vi "vi.Array2Array.vi"(0 "Array":variant[](array[variant]), 11 "error in (no error)":errorcluster) -> (4 "ClusterArray":variant, 15 "error out":errorcluster)   [LabVIEW 2014, in "GLue.lvlib" / "class.GLue.lvclass"]
uses:
  class.GLue.lvclass
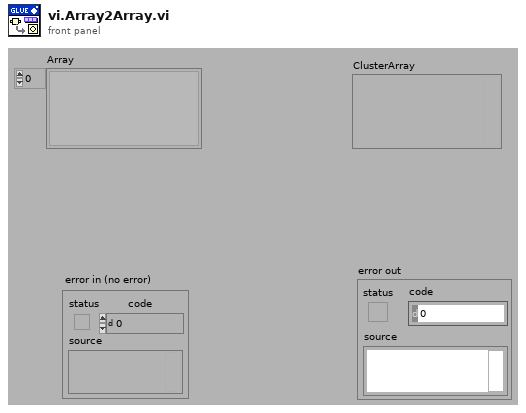
[diagram p1: front panel]
types:
  T1 = enum8{"<Null>", "I8", "I16", "I32", "I64", "U8", "U16", "U32", "U64", "SGL", "DBL", "EXT", "CSG", "CDB", "CXT", "0x0F", "0x10", "0x11", "0x12", "0x13", "0x14", "Enum U8", "Enum U16", "Enum U32", "Enum U64", "SGL PQ", "DBL PQ", "EXT PQ", "CSG PQ", "CDB PQ", "CXT PQ", "0x1F", "0x20", "Boolean", "0x22", "0x23", "0x24", "0x25", "0x26", "0x27", "0x28", "0x29", "0x2A", "0x2B", "0x2C", "0x2D", "0x2E", "0x2F", "String", "0x31", "Path", "Pict", "0x34", "0x35", "0x36", "DAQ", "0x38", "0x39", "0x3A", "0x3B", "0x3C", "0x3D", "0x3E", "0x3F", "Array", "0x41", "0x42", "0x43", "0x44", "0x45", "0x46", "0x47", "0x48", "0x49", "0x4A", "0x4B", "0x4C", "0x4D", "0x4E", "0x4F", "Cluster", "0x51", "0x52", "Variant", "Waveform", "0x55", "0x56", "0x57", "0x58", "0x59", "0x5A", "0x5B", "0x5C", "0x5D", "0x5E", "0x5F", "0x60", "0x61", "0x62", "0x63", "0x64", "0x65", "0x66", "0x67", "0x68", "0x69", "0x6A", "0x6B", "0x6C", "0x6D", "0x6E", "0x6F", "Refnum"}
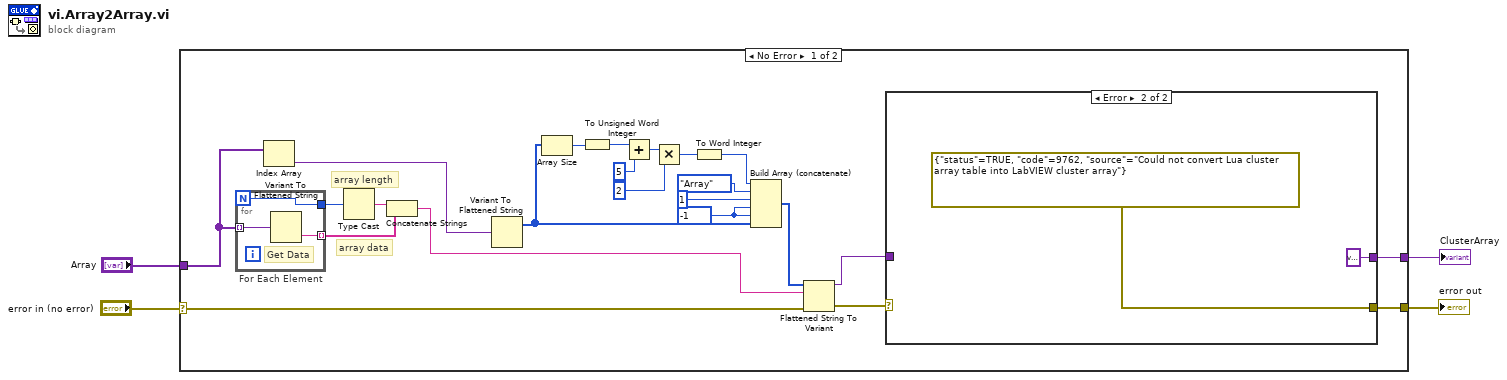
[diagram p0: block diagram]
diagram:
  n1 = case shown="No Error" "error in (no error)" {
    selector: "error in (no error)" -> [w9 w35]
    tunnel: "Array" -> [w24 _]
    tunnel: [w5 variant ("Variant")] -> w1
    tunnel: [w6 w35] -> w2
    frame No Error {
      w14 = i16 -1
      # "array length"
      # "array data"
      n2 = for "For Each Element" {
        N -> [w32]
        tunnel: w24 -> [w34] mode=indexing
        tunnel: [w33] -> w25 mode=indexing
        tunnel: [w32] -> w27
        # "Get Data"
        n3 = Variant To Flattened String(Variant=w34) -> (data string=w33:string)  [unwired: 1 out]
      }
      n4 = Index Array(array=w24) -> (element=w11:variant)  [unwired: 1 in]
      n5 = Type Cast(x=w27) -> (*(type *) &x=w26:string)  [unwired: 1 in]
      n6 = Concatenate Strings(w26, w25) -> (w10:string)
      n7 = Variant To Flattened String(Variant=w11) -> (1:w16:i16[])  [unwired: 1 out]
      n8 = Array Size(array=w16) -> (size(s)=w17:i32)
      n9 = To Unsigned Word Integer(number=w17) -> (unsigned 16bit integer=w19:u16)
      n10 = Add(x=w19, y=u16 5) -> (x+y=w21:u16)
      n11 = Multiply(x=w21, y=u16 2) -> (x*y=w23:u16)
      n12 = To Word Integer(number=w23) -> (16bit integer=w18:i16)
      n13 = Build Array (concatenate)(w18, T1."Array", i16 1, w14, w14, w16) -> (w12:i16[])
      n14 = Flattened String To Variant(4:w9, 6:w10, 7:w12) -> (0:w8:errorcluster, 3:w7:variant)
      n15 = case shown="Error" w8 {
        selector: w8 -> [w29 _]
        tunnel: w7 -> [w28 _]
        tunnel: [w29 errorcluster {"status"=TRUE, "code"=9762, "source"="Could not convert Lua cluster array table into LabVIEW cluster array"} ("error IO")] -> w6
        tunnel: [w28 variant ("Variant")] -> w5
        frame No Error {
        }
        frame Error {
        }
      }
    }
    frame Error {
    }
  }
  "error out" <- w2
  "ClusterArray" <- w1
